vi "Delete Child Items.vi"(8 "error in (no error)":errorcluster, 10 "Item Edit":string, 11 "TreeControl in":refnum<vi>) -> (0 "error out":errorcluster, 3 "TreeControl out":refnum<vi>)   [LabVIEW 2021]
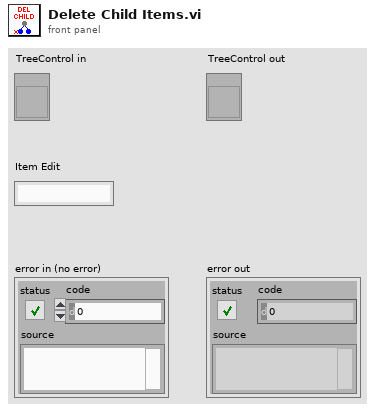
[diagram p1: front panel]
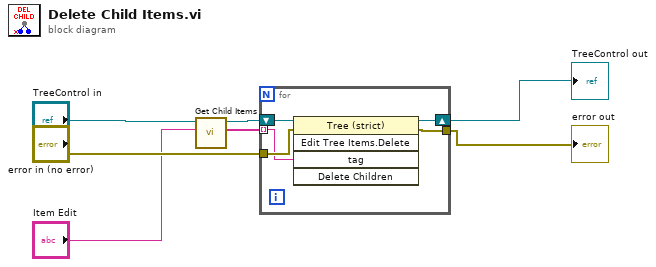
[diagram p0: block diagram]
diagram:
  n1 = call "Get Child Items.vi"("Node"="Item Edit", "TreeControl in"="TreeControl in") -> ("Child Array"=w7:string[], "TreeControl out"=w6:refnum<vi>)  [unwired: 8 in]
  n2 = for {
    shift-right: [w12] -> w3
    shift-left: w6 -> [w9]
    tunnel: "error in (no error)" -> [w11]
    tunnel: [w10] -> w5
    tunnel: w7 -> [w8] mode=indexing
    n3 = invoke class="Tree (strict)" method="Edit Tree Items.Delete"(reference=w9, error in=w11, "tag"=w8) -> (reference out=w12:refnum<vi>, error out=w10:errorcluster)  [unwired: 2 in, 3 out]
  }
  "error out" <- w5
  "TreeControl out" <- w3
